vi "CameraShutdown.vi"(1 "error in (no error)":errorcluster) -> (0 "error out":errorcluster)   [LabVIEW 2019]
uses:
  <userlib>/atmcd32d.llb/Error Code Enum typedef.ctl
  <userlib>/atmcd32d.llb/Shutter_mode typedef.ctl
  <userlib>/atmcd32d.llb/Shutter_type typedef.ctl
panel:
  out "Camera OK?":bool
  out "Numeric":i32
  out "Cooler DLL error code 2":u32
  out "DLL error code":u32
  out "status":T1
  out "Abort DLL error code":u32
  out "Temperature":i32
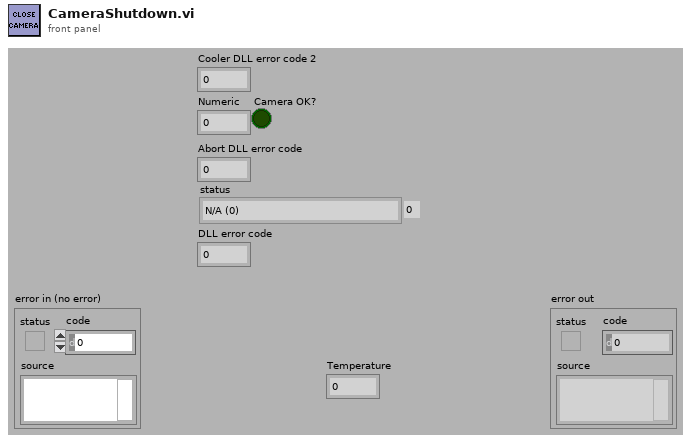
[diagram p1: front panel]
types:
  T1 = typedef "Error Code Enum typedef.ctl" = enum32{"N/A (0)", "DRV_ERROR_CODES", "DRV_SUCCESS", "DRV_VXDNOTINSTALLED", "DRV_ERROR_SCAN", "DRV_ERROR_CHECK_SUM", "DRV_ERROR_FILELOAD", "DRV_UNKNOWN_FUNC", "DRV_ERROR_VXD_INIT", "DRV_ERROR_ADDRESS", "DRV_ERROR_PAGELOCK", "DRV_ERROR_PAGEUNLOCK", "DRV_ERROR_BOARDTEST", "DRV_ERROR_ACK", "DRV_ERROR_UP_FIFO", "DRV_ERROR_PATTERN", "N/A (16)", "DRV_ACQUISITION_ERRORS", "DRV_ACQ_BUFFER", "DRV_ACQ_DOWNFIFO_FULL", "DRV_PROC_UNKONWN_INSTRUCTION", "DRV_ILLEGAL_OP_CODE", "DRV_KINETIC_TIME_NOT_MET", "DRV_ACCUM_TIME_NOT_MET", "DRV_NO_NEW_DATA", "N/A (25)", "DRV_SPOOLERROR", "N/A (27)", "N/A (28)", "N/A (29)", "N/A (30)", "N/A (31)", "N/A (32)", "DRV_TEMPERATURE_CODES", "DRV_TEMPERATURE_OFF", "DRV_TEMPERATURE_NOT_STABILIZED", "DRV_TEMPERATURE_STABILIZED", "DRV_TEMPERATURE_NOT_REACHED", "DRV_TEMPERATURE_OUT_RANGE", "DRV_TEMPERATURE_NOT_SUPPORTED", "DRV_TEMPERATURE_DRIFT", "N/A (41)", "N/A (42)", "N/A (43)", "N/A (44)", "N/A (45)", "N/A (46)", "N/A (47)", "N/A (48)", "DRV_GENERAL_ERRORS", "DRV_INVALID_AUX", "DRV_COF_NOTLOADED", "DRV_FPGAPROG", "DRV_FLEXERROR", "DRV_GPIBERROR", "N/A (55)", "N/A (56)", "N/A (57)", "N/A (58)", "N/A (59)", "N/A (60)", "N/A (61)", "N/A (62)", "N/A (63)", "DRV_DATATYPE", "DRV_DRIVER_ERRORS", "DRV_P1INVALID", "DRV_P2INVALID", "DRV_P3INVALID", "DRV_P4INVALID", "DRV_INIERROR", "DRV_COFERROR", "DRV_ACQUIRING", "DRV_IDLE", "DRV_TEMPCYCLE", "DRV_NOT_INITIALIZED", "DRV_P5INVALID", "DRV_P6INVALID", "DRV_INVALID_MODE", "DRV_INVALID_FILTER", "DRV_I2CERRORS", "DRV_I2CDEVNOTFOUND", "DRV_I2CTIMEOUT", "DRV_P7INVALID", "N/A (84)", "N/A (85)", "N/A (86)", "N/A (87)", "N/A (88)", "N/A (89)", "DRV_IOCERROR", "DRV_VRMVERSIONERROR"}
  T2 = typedef "Shutter_type typedef.ctl" = enum16{"TTL Low", "TTL High"}
  T3 = typedef "Shutter_mode typedef.ctl" = enum16{"Auto", "Open", "Close", "N/A (3)", "Open FVB Series", "Open Any Series"}
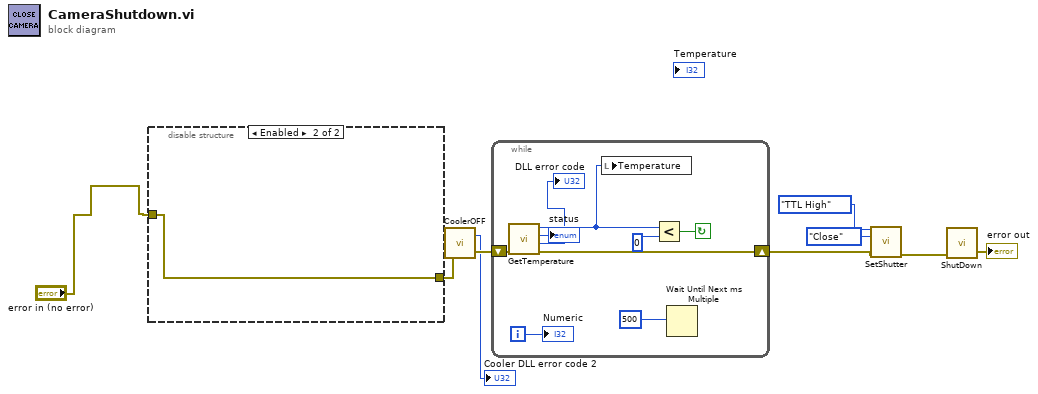
[diagram p0: block diagram]
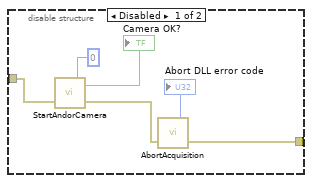
[diagram p2: hidden frame]
diagram:
  n1 = disable-structure shown="Enabled" {
    disable-tunnel: [w15 w16] -> w4
    disable-tunnel: "error in (no error)" -> [w12 w16]
    frame Disabled {
      n2 = call "StartAndorCamera.vi"("error in (no error)"=w12, "Initial temp"=0) -> ("error out"=w10:errorcluster, "Camera OK?"=→"Camera OK?":bool)
      n3 = call <userlib>:"AbortAcquisition.vi"("error in (no error)"=w10) -> ("error out"=w15:errorcluster, "DLL error code"=→"Abort DLL error code":u32)  [unwired: 1 in]
    }
    frame Enabled {
    }
  }
  n4 = call <userlib>:"CoolerOFF.vi"("error in (no error)"=w4) -> ("error out"=w9:errorcluster, "DLL error code"=→"Cooler DLL error code 2":u32)  [unwired: 1 in]
  n5 = while {
    shift-right: [w21] -> w8
    shift-left: w9 -> [w22]
    i -> [w17]
    stop <- w24 continue-if-true
    n6 = call <userlib>:"GetTemperature.vi"("error in (no error)"=w22) -> ("error out"=w21:errorcluster, "DLL error code"=→"DLL error code":u32, "status"=→"status":T1, "temperature"=w20:i32)  [unwired: 3 in]
    n7 = local write "Temperature"(w20) -> ()
    n8 = Less?(x=w20, y=0) -> (x < y?=w24:bool)
    n9 = Wait Until Next ms Multiple(millisecond multiple=u32 500) -> ()  [unwired: 1 out]
    "Numeric" <- w17
  }
  n10 = call <userlib>:"SetShutter.vi"("type"=Shutter_type_typedef."TTL High", "mode"=Shutter_mode_typedef."Close", "error in (no error)"=w8) -> ("error out"=w7:errorcluster)  [unwired: 11 in, 1 out]
  n11 = call <userlib>:"ShutDown.vi"("error in (no error)"=w7) -> ("error out"=→"error out":errorcluster)  [unwired: 1 in, 1 out]
